vi "ArrayToTable(SubVI).vi"(9 "Telemetry":T1=[{"ID"="", "Num"=0, "Name"="", "Desc"="", "Unit"="", "FormatStr"="", "Min"=0, "Max"=0}], 11 "Data in":sgl[](array[numeric])) -> (3 "Table out":string[][](array[string]))   [LabVIEW 2017, in "LV_Unicorn.lvlib"]
uses:
  LV_Unicorn.lvlib
  Control/unicorn_Telemetry.ctl
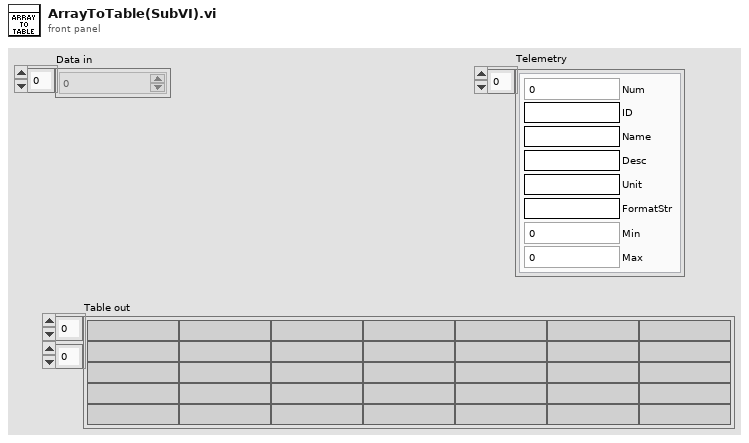
[diagram p1: front panel]
types:
  T1 = typedef "LV_Unicorn.lvlib/unicorn_Telemetry.ctl" = cluster{"ID":string, "Num":i32, "Name":string, "Desc":string, "Unit":string, "FormatStr":string, "Min":i32, "Max":i32}[]
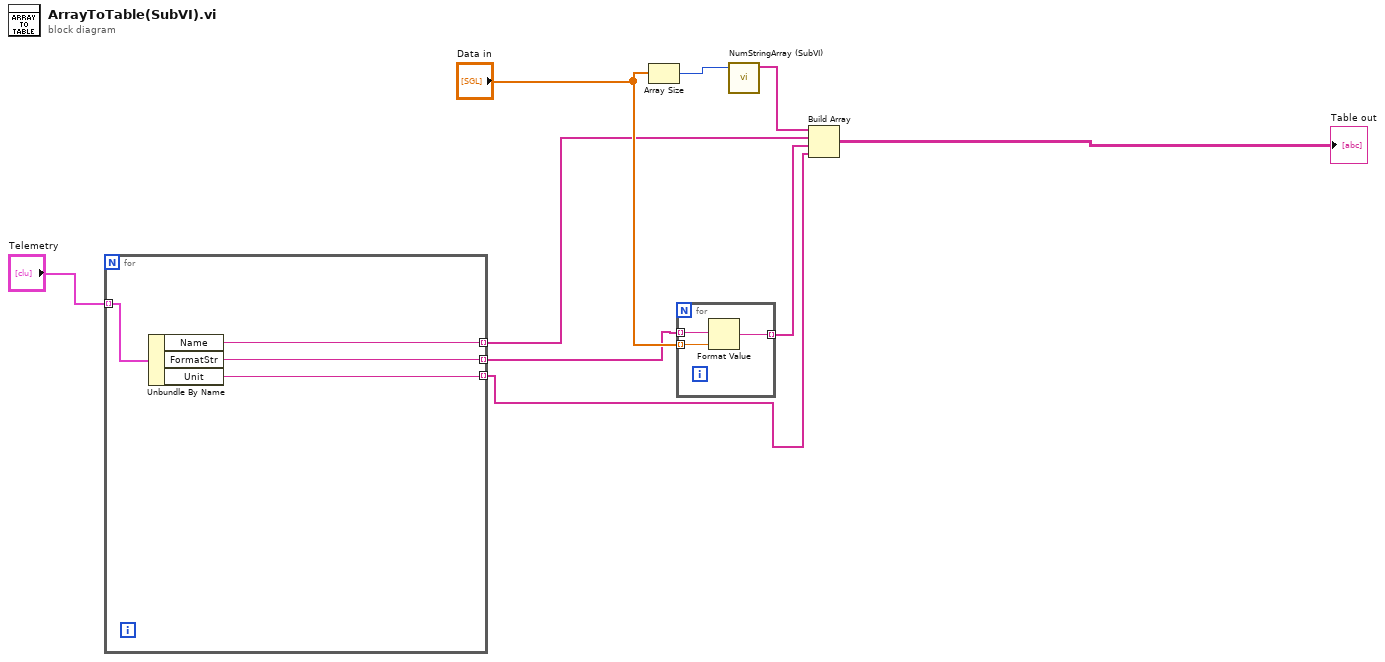
[diagram p0: block diagram]
diagram:
  n1 = for {
    tunnel: "Telemetry" -> [w13] mode=indexing
    tunnel: [w12] -> w3 mode=indexing
    tunnel: [w11] -> w2 mode=indexing
    tunnel: [w10] -> w1 mode=indexing
    n2 = Unbundle By Name(w13) -> ("Name"=w12:string, "FormatStr"=w11:string, "Unit"=w10:string)
  }
  n3 = Array Size(array="Data in") -> (size(s)=w8:i32)
  n4 = for {
    tunnel: "Data in" -> [w16] mode=indexing
    tunnel: [w15] -> w7 mode=indexing
    tunnel: w2 -> [w14] mode=indexing
    n5 = Format Value(format string=w14, value (0)=w16) -> (output string=w15:string)  [unwired: 1 in]
  }
  n6 = call "NumStringArray (SubVI).vi"("NInt"=w8) -> ("Array"=w5:string[])  [unwired: 10 in]
  n7 = Build Array(w5, w3, w7, w1) -> (→"Table out":string[][])
